vi "Word Count.vi"() -> ()   [LabVIEW 2017]
panel:
  out "Output":string
  out "Word Count":dbl
  in  "Word":string
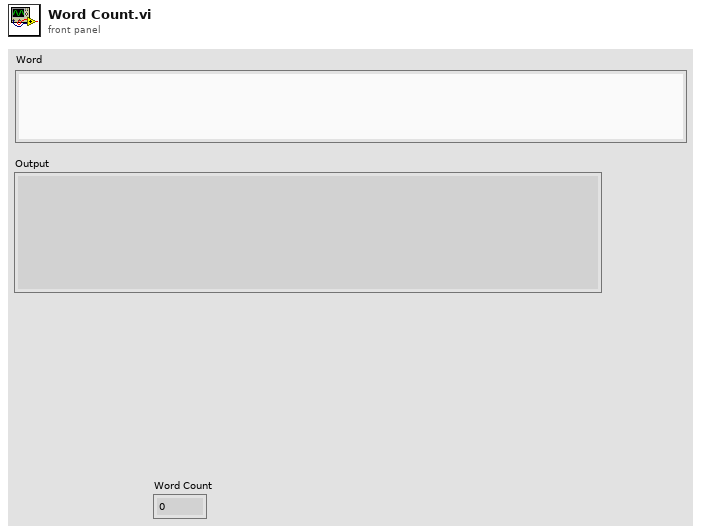
[diagram p1: front panel]
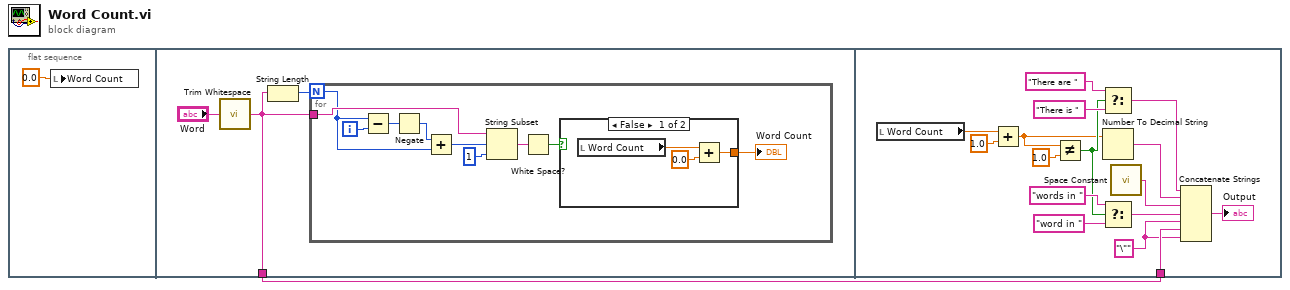
[diagram p0: block diagram]
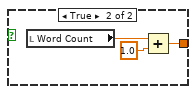
[diagram p2: hidden frame]
diagram:
  n1 = flat-sequence {
    tunnel: [w3] -> w1
    tunnel: w1 -> [w23]
    frame #0 {
      n2 = local write "Word Count"(0.0 ("Word Count")) -> ()
    }
    frame #1 {
      n3 = call <vilib>:"Trim Whitespace.vi"("string"="Word") -> ("trimmed string"=w3:string)  [unwired: 1 in]
      n4 = String Length(string=w3) -> (length=w5:i32)
      n5 = for {
        N: w5 -> [w9]
        tunnel: w3 -> [w15]
        i -> [w6]
        n6 = Subtract(x=w9, y=w6) -> (x-y=w11:i32)
        n7 = Negate(x=w11) -> (-x=w10:i32)
        n8 = Add(x=w10, y=w9) -> (x+y=w8:i32)
        n9 = String Subset(string=w15, offset (0)=w8, length (rest)=1 ("length (rest)")) -> (substring=w12:string)
        n10 = White Space?(1:w12) -> (0:w13:bool)
        n11 = case shown="False" w13 {
          tunnel: [w16 w20] -> w7
          frame False {
            n12 = local read "Word Count"() -> (w18:dbl)
            n13 = Add(x=w18, y=0.0) -> (x+y=w16:dbl)
          }
          frame True {
            n14 = local read "Word Count"() -> (w21:dbl)
            n15 = Add(x=w21, y=1.0) -> (x+y=w20:dbl)
          }
        }
        "Word Count" <- w7
      }
    }
    frame #2 {
      w22 = "\"" ("string")
      n16 = local read "Word Count"() -> (w26:dbl)
      n17 = Add(x=w26, y=1.0) -> (x+y=w25:dbl)
      n18 = Not Equal?(x=w25, y=1.0) -> (x != y?=w29:bool)
      n19 = Select(t="There are " ("string"), s=w29, f="There is ") -> (s? t:f=w28:string)
      n20 = Number To Decimal String(number=w25) -> (decimal integer string=w37:string)  [unwired: 1 in]
      n21 = Select(t="words in ", s=w29, f="word in ") -> (s? t:f=w31:string)
      n22 = call <vilib>:"Space Constant.vi"() -> ("String"=w33:string)
      n23 = Concatenate Strings(w28, w37, w33, w31, w22, w23, w22) -> (→"Output":string)
    }
  }
